vi "Deserialize (Byte Array).vi"(8 "error in (no error)":errorcluster, 10 "Serialized":i8[](array[numeric]), 11 "Data in":refnum<class "Data.lvclass">) -> (0 "error out":errorcluster, 2 "Returned data out":refnum<class "Data.lvclass">, 3 "Data out":refnum<class "Data.lvclass">)   [LabVIEW 2015, in "MDSplus.lvlib" / "Data.lvclass"]
uses:
  Data.lvclass
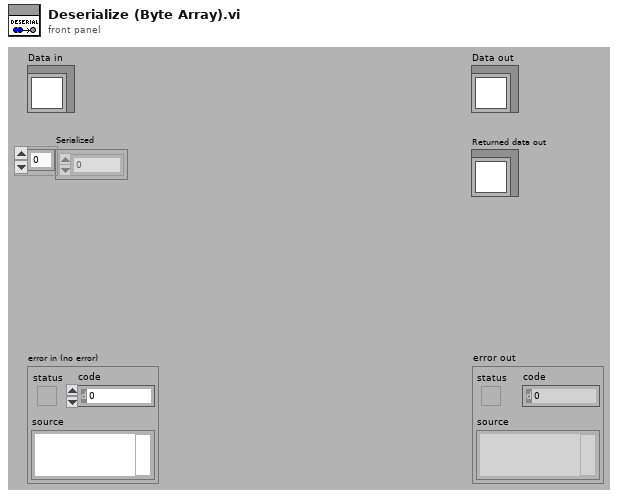
[diagram p1: front panel]
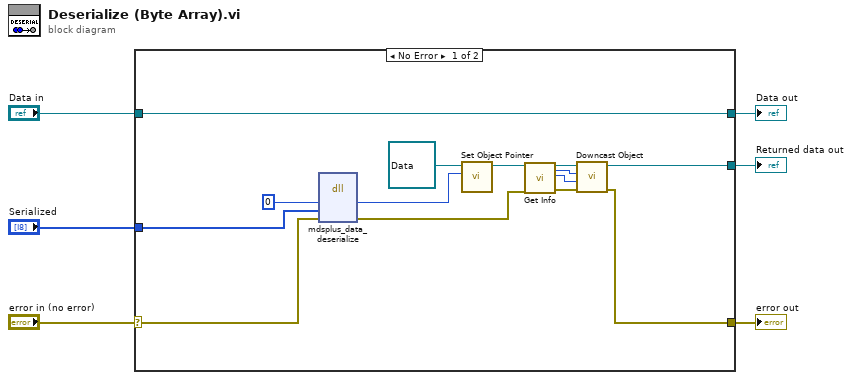
[diagram p0: block diagram]
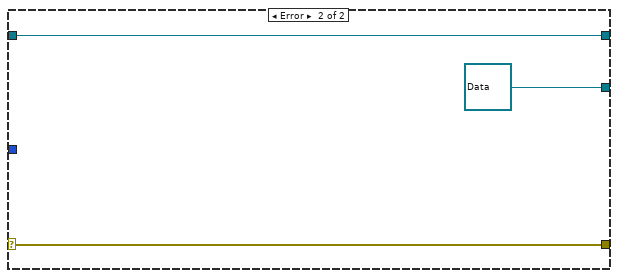
[diagram p2: hidden frame]
diagram:
  n1 = case shown="No Error" "error in (no error)" {
    selector: "error in (no error)" -> [w19 w23]
    tunnel: [w9 w23] -> w5
    tunnel: "Serialized" -> [w20 _]
    tunnel: [w8 refnum<class "Data.lvclass"> refnum ("MDSplus.lvlib:Data.lvclass")] -> w3
    tunnel: [w7 w21] -> w1
    tunnel: "Data in" -> [w7 w21]
    frame No Error {
      n2 = dll-call lib="MDSobjectsLVShr" fn="mdsplus_data_deserialize"("lvDataPtrOut"=i64 0 ("lvTreeNodePtr"), "serializedIn"=w20, "error"=w19) -> ("lvDataPtrOut"=w11:i64, "error"=w10:errorcluster)  [unwired: 5 in, 2 out]
      n3 = call-dynamic "Set Object Pointer.vi"("Object Pointer"=w11, "Data in"=refnum<class "Data.lvclass"> refnum ("Data.lvclass")) -> ("Data out"=w16:refnum<class "Data.lvclass">)  [unwired: 9 in]
      n4 = call-dynamic "Get Info.vi"("Data in"=w16, "error in (no error)"=w10) -> ("Data out"=w15:refnum<class "Data.lvclass">, "Class type out"=w14:u8, "Data type out"=w13:u8, "error out"=w12:errorcluster)  [unwired: 12 in, 2 out]
      n5 = call "Downcast Object.vi"("error in (no error)"=w12, "Data Type"=w13, "Class Type"=w14, "Data in"=w15) -> ("error out"=w9:errorcluster, "Data out"=w8:refnum<class "Data.lvclass">)  [unwired: 6 in]
    }
    frame Error {
    }
  }
  "error out" <- w5
  "Returned data out" <- w3
  "Data out" <- w1
